vi "FPGA Settings.vi"(8 "error in":errorcluster, 9 "Action":T2, 10 "FPGA Settings":T1={"Bitfile path"=path "", "RIO Device Address"="RIO0", "Group"=FALSE}, 11 "VS Engine Interface in":refnum<class "VS Engine Interface.lvclass">) -> (0 "error out":errorcluster, 2 "FPGA Settings":T1, 3 "VS Engine Interface out":refnum<class "VS Engine Interface.lvclass">)   [LabVIEW 2024, in "VS Engine Abstraction.lvlib" / "VS Engine Interface.lvclass"]
uses:
  VS Engine Interface.lvclass
  Addon Shared/Types/FPGA Settings.ctl
  Addon Shared/FPGA Addon Shared.lvlib
  Addon Shared/Types/FG Action.ctl
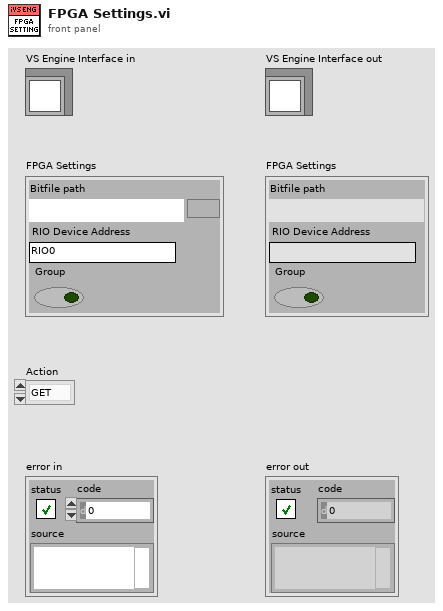
[diagram p1: front panel]
types:
  T1 = typedef "FPGA Addon Shared.lvlib/FPGA Settings.ctl" = cluster{"Bitfile path":path, "RIO Device Address":string, "Group":bool}
  T2 = typedef "FPGA Addon Shared.lvlib/FG Action.ctl" = enum8{"GET", "SET"}
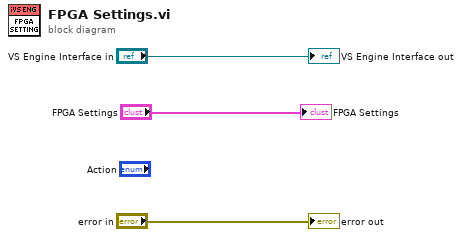
[diagram p0: block diagram]
diagram:
  "error out" <- "error in"
  "VS Engine Interface out" <- "VS Engine Interface in"
  "FPGA Settings" <- "FPGA Settings"
